vi "Esophageal_Datalogger_ThresholdUpdated.vi"(8 "error in":errorcluster, 9 "MTN Threshold":dbl, 10 "Log File In":refnum<file>) -> (0 "error out":errorcluster, 2 "Log File Out":refnum<file>)   [LabVIEW 2021]
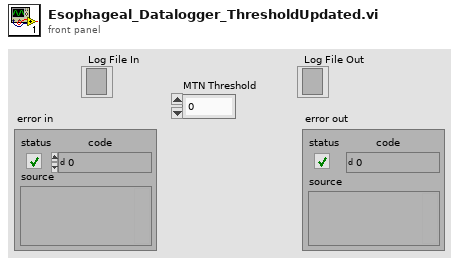
[diagram p1: front panel]
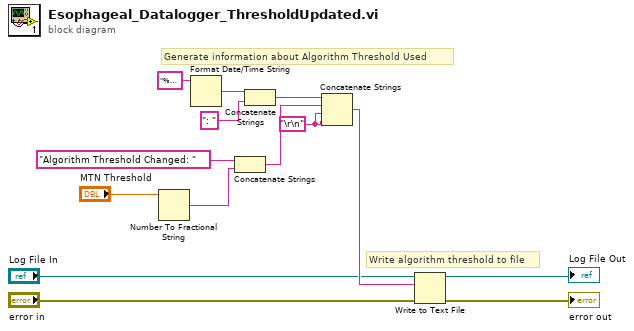
[diagram p0: block diagram]
diagram:
  w5 = "\r\n"
  # "Generate information about Algorithm Threshold Used"
  # "Write algorithm threshold to file"
  n1 = Number To Fractional String(number="MTN Threshold") -> (F-format string=w8:string)  [unwired: 3 in]
  n2 = Format Date/Time String(time format string (%c)="%H%M%S%3u") -> (date/time string=w10:string)  [unwired: 2 in]
  n3 = Concatenate Strings("Algorithm Threshold Changed: " ("time format string (%c)"), w8) -> (w14:string)
  n4 = Concatenate Strings(w10, ": " ("string")) -> (w12:string)
  n5 = Concatenate Strings(w12, w14, w5, w5) -> (w6:string)
  n6 = Write to Text File(file (use dialog)="Log File In", text=w6, error in="error in") -> (refnum out=→"Log File Out":refnum<file>, error out=→"error out":errorcluster)  [unwired: 1 in, 1 out]
